vi "Create Sysdef Tree from DB Channel Clusters_BC.vi"(7 "Autocreate Rx timestamp chans?":bool, 8 "error in":errorcluster, 10 "BC":T1, 11 "Device Ptr":u64) -> (0 "error out":errorcluster, 3 "Device Ptr dup":u64)   [LabVIEW 2020, in "Ballard 1553 System Explorer.lvlib"]
uses:
  Ballard 1553 System Explorer.lvlib
  Parse XML Ballard/Ballard_BC.ctl
  Parse XML Ballard/Ballard_message.ctl
  Parse XML Ballard/Ballard_messageType.ctl
  Parse XML Ballard/Ballard_CWD1.ctl
  Parse XML Ballard/Ballard_CWD2.ctl
  Parse XML Ballard/Ballard_minorFrame.ctl
  Parse XML Ballard/Ballard_majorFrame.ctl
  Parse XML Ballard/Ballard_acyclicFrame.ctl
  <vilib>/NI VeriStand/Custom Device API/Custom Device Channel.ctl
  <vilib>/NI VeriStand/Custom Device API/Custom Device Channel Type.ctl
  Shared/Controls and Global/Global.vi
  <userlib>/_OpenG.lib/array/array.llb/Remove Duplicates from 1D Array (I32)__ogtk.vi
  <vilib>/NI VeriStand/Custom Device API/Set Item Property (String).vi
  <vilib>/NI VeriStand/Custom Device API/Set Item Property (U16).vi
  <vilib>/NI VeriStand/Custom Device API/Set Item Property (Variant).vi
  <vilib>/NI VeriStand/Custom Device API/Set Item Property (I32).vi
  <vilib>/NI VeriStand/Custom Device API/Custom Device API.lvlib
  Shared/Ballard 1553 Shared.lvlib
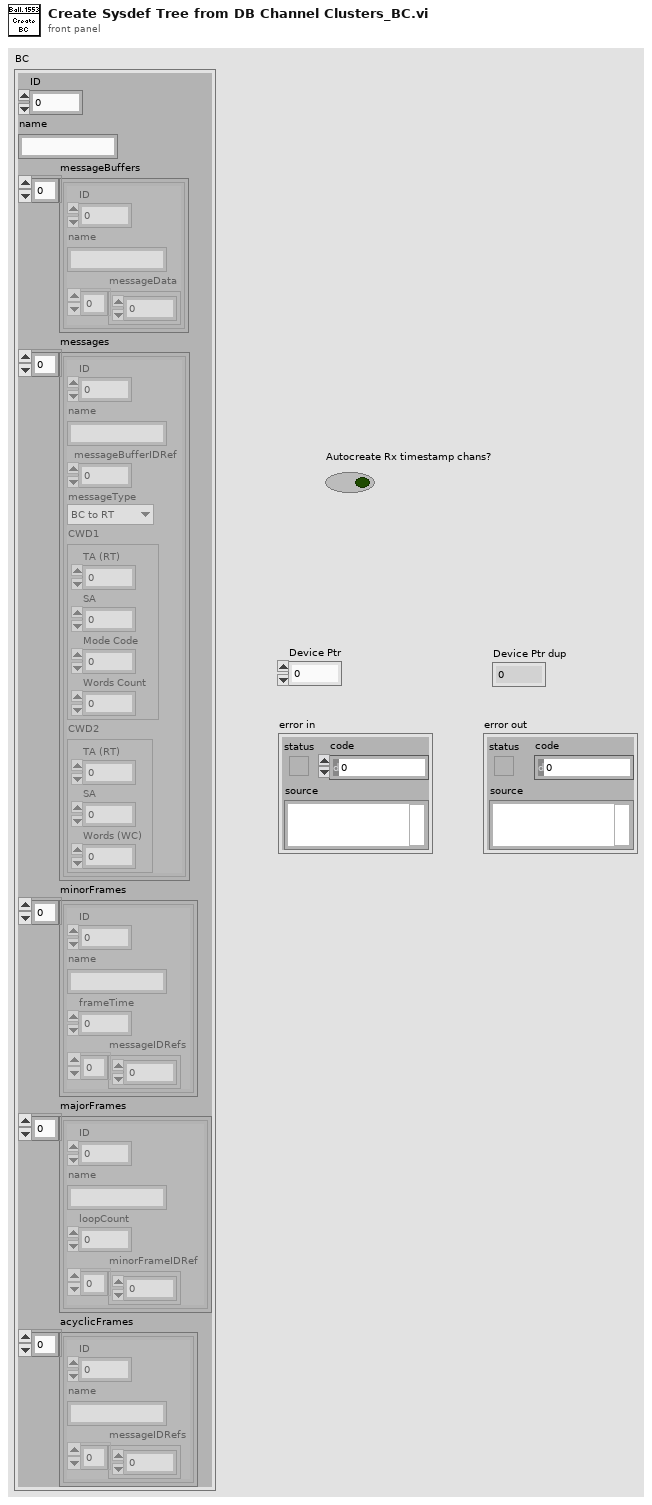
[diagram p1: front panel]
types:
  T1 = typedef "Ballard 1553 System Explorer.lvlib/Ballard_BC.ctl" = cluster{"ID":i32, "name":string, "messageBuffers":cluster{"ID":i32, "name":string, "messageData":u16[]}[], "messages":T2[], "minorFrames":T6[], "majorFrames":T7[], "acyclicFrames":T8[]}
  T2 = typedef "Ballard 1553 System Explorer.lvlib/Ballard_message.ctl" = cluster{"ID":i32, "name":string, "messageBufferIDRef":i32, "messageType":T3, "CWD1":T4, "CWD2":T5}
  T3 = typedef "Ballard 1553 System Explorer.lvlib/Ballard_messageType.ctl" = enum16{"BC to RT", "RT to BC", "RT to RT", "MC (Rx)", "MC (Tx)"}
  T4 = typedef "Ballard 1553 System Explorer.lvlib/Ballard_CWD1.ctl" = cluster{"TA (RT)":i8, "SA":i8, "Mode Code":i8, "Words Count":i8}
  T5 = typedef "Ballard 1553 System Explorer.lvlib/Ballard_CWD2.ctl" = cluster{"TA (RT)":i8, "SA":i8, "Words (WC)":i8}
  T6 = typedef "Ballard 1553 System Explorer.lvlib/Ballard_minorFrame.ctl" = cluster{"ID":i32, "name":string, "frameTime":i32, "messageIDRefs":i32[]}
  T7 = typedef "Ballard 1553 System Explorer.lvlib/Ballard_majorFrame.ctl" = cluster{"ID":i32, "name":string, "loopCount":i32, "minorFrameIDRef":i32[]}
  T8 = typedef "Ballard 1553 System Explorer.lvlib/Ballard_acyclicFrame.ctl" = cluster{"ID":i32, "name":string, "messageIDRefs":i32[]}
  T9 = typedef "Custom Device API.lvlib/Custom Device Channel.ctl" = cluster{"Type":T10, "Units":string, "Default Value":dbl, "Faultable":bool, "Scalable":bool}
  T10 = typedef "Custom Device API.lvlib/Custom Device Channel Type.ctl" = enum16{"Input", "Output"}
  T11 = cluster{"ID":i32, "name":string, "messageData":u16[]}[]
  T12 = typedef "Custom Device API.lvlib/Custom Device Item Ref.ctl" = u64
  T13 = cluster{"ID":i32, "name":string, "messageData":u16[]}
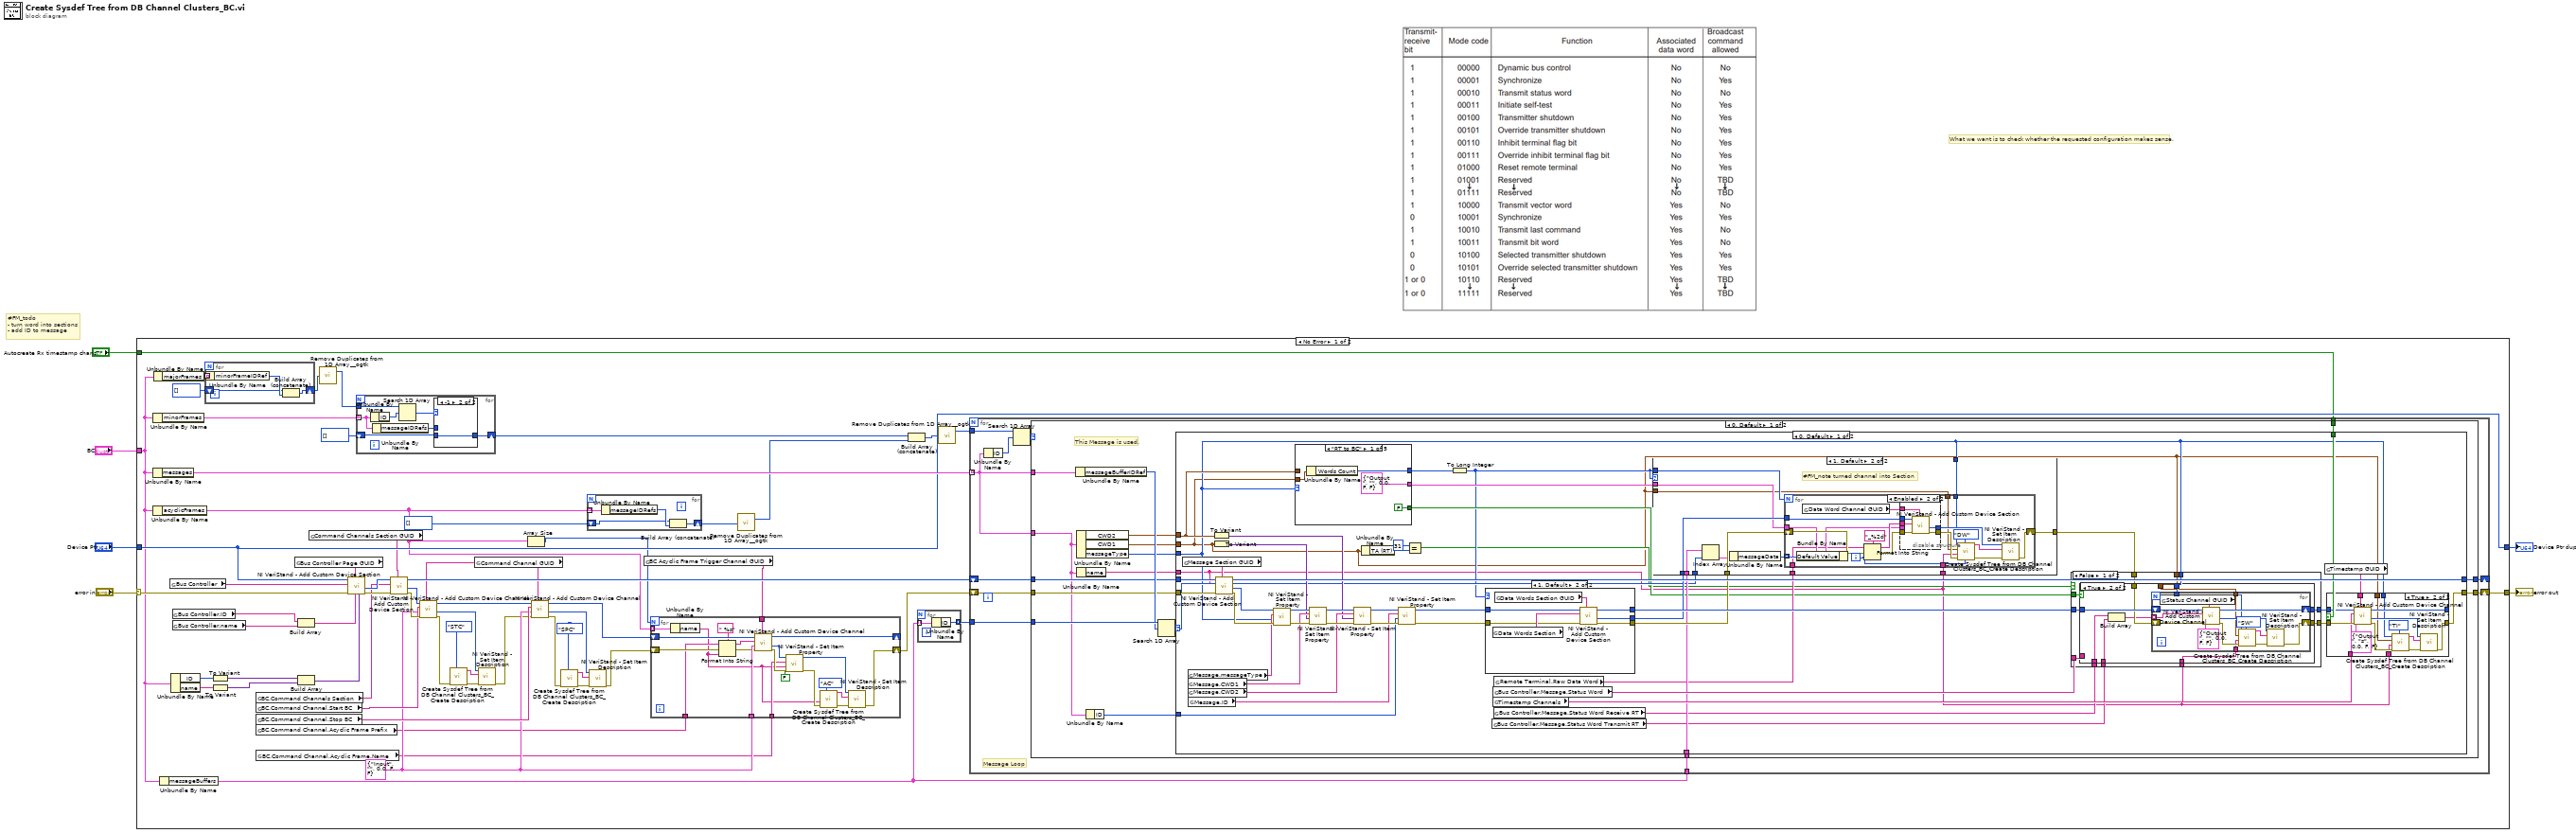
[diagram p0: block diagram]
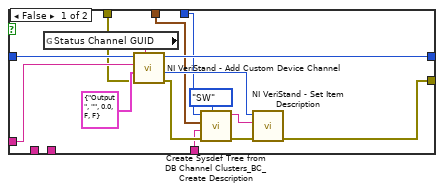
[diagram p2: hidden frame]
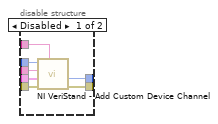
[diagram p6: hidden frame]
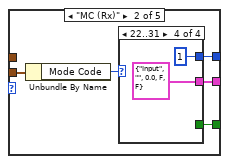
[diagram p7: hidden frame]
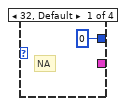
[diagram p8: hidden frame]
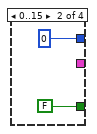
[diagram p9: hidden frame]
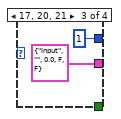
[diagram p10: hidden frame]
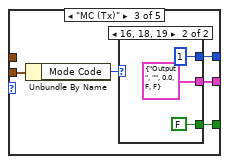
[diagram p11: hidden frame]
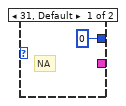
[diagram p12: hidden frame]
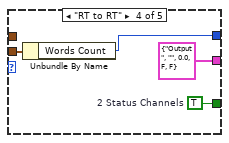
[diagram p13: hidden frame]
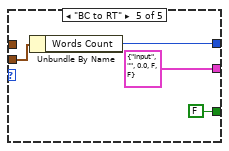
[diagram p14: hidden frame]
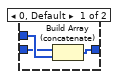
[diagram p18: hidden frame]
diagram:
  # "#FM_todo \n- turn word into sections\n- add ID to message"
  # "What we want is to check whether the requested configuration makes sense."
  n1 = case shown="No Error" "error in" {
    selector: "error in" -> [w67 w349]
    tunnel: [w49 w349] -> w5
    tunnel: "Device Ptr" -> [w50 w348]
    tunnel: [w50 w348] -> w3
    tunnel: "BC" -> [w34 _]
    tunnel: "Autocreate Rx timestamp chans?" -> [w46 _]
    frame No Error {
      w25 = T9 {"Type"=enum."Input", "Units"="", "Default Value"=0.0, "Faultable"=FALSE, "Scalable"=FALSE} ("Channel")
      n2 = Unbundle By Name(w34) -> ("minorFrames"=w57:T6[])
      n3 = Unbundle By Name(w34) -> ("messages"=w54:T2[])
      n4 = Unbundle By Name(w34) -> ("acyclicFrames"=w23:T8[])
      n5 = Unbundle By Name(w34) -> ("majorFrames"=w58:T7[])
      n6 = Unbundle By Name(w34) -> ("messageBuffers"=w52:T11)
      n7 = global read "Global.vi" "Bus Controller"() -> (w65:string)
      n8 = Unbundle By Name(w34) -> ("ID"=w64:i32, "name"=w63:string)
      n9 = global read "Global.vi" "Bus Controller.ID"() -> (w36:string)
      n10 = global read "Global.vi" "Bus Controller.name"() -> (w35:string)
      n11 = for {
        tunnel: w58 -> [w347] mode=indexing
        shift-right: [w346] -> w47
        shift-left: i32[] [] -> [w344]
        n12 = Unbundle By Name(w347) -> ("minorFrameIDRef"=w345:i32[])
        n13 = Build Array (concatenate)(w344, w345) -> (w346:i32[])
      }
      n14 = To Variant(anything=w64) -> (Variant=w62:variant)
      n15 = To Variant(anything=w63) -> (Variant=w61:variant)
      n16 = global read "Global.vi" "BC.Command Channels Section"() -> (w39:string)
      n17 = global read "Global.vi" "BC.Command Channel.Start BC"() -> (w38:string)
      n18 = global read "Global.vi" "BC.Command Channel.Stop BC"() -> (w37:string)
      n19 = global read "Global.vi" "BC.Command Channel.Acyclic Frame Prefix"() -> (w22:string)
      n20 = global read "Global.vi" "BC.Command Channel.Acyclic Frame.Name"() -> (w19:string)
      n21 = global read "Global.vi" "Bus Controller Page GUID"() -> (w66:string)
      n22 = Build Array(w36, w35) -> (w60:string[])
      n23 = Build Array(w62, w61) -> (w59:variant[])
      n24 = global read "Global.vi" "Command Channels Section GUID"() -> (w20:string)
      n25 = call-poly <userlib>:"Remove Duplicates from 1D Array__ogtk.vi"("Input Array"=w47) -> ("Output Array"=w56:i32[])  [unwired: 1 out]
      n26 = call <vilib>:"NI VeriStand - Add Custom Device Section.vi"("Property Values"=w59, "Property names"=w60, "GUID (Default Section)"=w66, "error in (no error)"=w67, "Section Name"=w65, "Parent Ref in"=w50) -> ("error out"=w40:errorcluster, "Section Ptr"=w42:T12)  [unwired: 2 in, 2 out]
      n27 = for {
        tunnel: w57 -> [w336] mode=indexing
        tunnel: w56 -> [w339]
        shift-right: [w334] -> w31
        shift-left: i32[] [] -> [w333]
        n28 = Unbundle By Name(w336) -> ("ID"=w338:i32)
        n29 = Unbundle By Name(w336) -> ("messageIDRefs"=w335:i32[])
        n30 = Search 1D Array(1D array=w339, element=w338) -> (index of element=w337:i32)  [unwired: 1 in]
        n31 = case shown="-1" w337 {
          tunnel: w335 -> [w342 _]
          tunnel: [w341 w343] -> w334
          tunnel: w333 -> [w340 w343]
          frame 0, Default {
            n32 = Build Array (concatenate)(w340, w342) -> (w341:i32[])
          }
          frame -1 {
          }
        }
      }
      n33 = call <vilib>:"NI VeriStand - Add Custom Device Section.vi"("GUID (Default Section)"=w20, "error in (no error)"=w40, "Section Name"=w39, "Parent Ref in"=w42) -> ("error out"=w44:errorcluster, "Section Ptr"=w43:T12, "Parent Ref out"=w41:T12)  [unwired: 4 in, 1 out]
      n34 = global read "Global.vi" "Command Channel GUID"() -> (w27:string)
      n35 = call <vilib>:"NI VeriStand - Add Custom Device Channel.vi"("GUID (Default Channel)"=w27, "error in (no error)"=w44, "Channel"=w25, "Channel Name"=w38, "Parent Ref in"=w43) -> ("error out"=w17:errorcluster, "Channel Ref"=w16:T12, "Parent Ref out"=w45:T12)  [unwired: 3 in, 1 out]
      n36 = call "Create Sysdef Tree from DB Channel Clusters_BC_Create Description.vi"("Type"=enum16{"DW", "STC", "SPC", "SW", "TI", "AC"}."STC", "error in (no error)"=w17) -> ("error out"=w14:errorcluster, "Description (Out)"=w18:string)  [unwired: 8 in]
      n37 = call <vilib>:"NI VeriStand - Set Item Description.vi"("error in (no error)"=w14, "Description"=w18, "Item Ref in"=w16) -> ("error out"=w15:errorcluster)  [unwired: 6 in, 2 out]
      n38 = Array Size(array=w23) -> (size(s)=w26:i32)
      n39 = call <vilib>:"NI VeriStand - Add Custom Device Channel.vi"("GUID (Default Channel)"=w27, "error in (no error)"=w15, "Channel"=w25, "Channel Name"=w37, "Parent Ref in"=w45) -> ("error out"=w10:errorcluster, "Channel Ref"=w8:T12, "Parent Ref out"=w24:T12)  [unwired: 3 in, 1 out]
      n40 = call "Create Sysdef Tree from DB Channel Clusters_BC_Create Description.vi"("Type"=enum16{"DW", "STC", "SPC", "SW", "TI", "AC"}."SPC", "error in (no error)"=w10) -> ("error out"=w12:errorcluster, "Description (Out)"=w11:string)  [unwired: 8 in]
      n41 = for {
        tunnel: w23 -> [w92] mode=indexing
        shift-right: [w90] -> w32
        shift-left: i32[] [] -> [w89]
        n42 = Unbundle By Name(w92) -> ("messageIDRefs"=w91:i32[])
        n43 = Build Array (concatenate)(w89, w91) -> (w90:i32[])
      }
      n44 = call <vilib>:"NI VeriStand - Set Item Description.vi"("error in (no error)"=w12, "Description"=w11, "Item Ref in"=w8) -> ("error out"=w9:errorcluster)  [unwired: 6 in, 2 out]
      n45 = global read "Global.vi" "BC Acyclic Frame Trigger Channel GUID"() -> (w21:string)
      n46 = for {
        N: w26 -> [_]
        shift-right: [w71] -> w28
        shift-left: w9 -> [w84]
        tunnel: w21 -> [w88]
        tunnel: w25 -> [w87]
        shift-right: [w85] -> _
        shift-left: w24 -> [w86]
        tunnel: w23 -> [w82] mode=indexing
        tunnel: w22 -> [w81]
        tunnel: w19 -> [w75]
        n47 = Unbundle By Name(w82) -> ("name"=w68:string)
        n48 = Format Into String(format string=" %s", initial string=w81, error in=w84, w68) -> (resulting string=w79:string, error out=w83:errorcluster)
        n49 = call <vilib>:"NI VeriStand - Add Custom Device Channel.vi"("GUID (Default Channel)"=w88, "error in (no error)"=w83, "Channel"=w87, "Channel Name"=w79, "Parent Ref in"=w86) -> ("error out"=w76:errorcluster, "Channel Ref"=w78:T12, "Parent Ref out"=w85:T12)  [unwired: 3 in, 1 out]
        n50 = call-poly <vilib>:"NI VeriStand - Set Item Property.vi"("Binary String (T)"=FALSE, "error in (no error)"=w76, "Value"=w68, "Property Name"=w75, "Item Ref in"=w78) -> ("error out"=w69:errorcluster, "Item Ref out"=w70:T12)  [unwired: 4 in, 1 out]
        n51 = call "Create Sysdef Tree from DB Channel Clusters_BC_Create Description.vi"("Type"=enum16{"DW", "STC", "SPC", "SW", "TI", "AC"}."AC", "error in (no error)"=w69, "Message Name"=w68) -> ("error out"=w73:errorcluster, "Description (Out)"=w72:string)  [unwired: 7 in]
        n52 = call <vilib>:"NI VeriStand - Set Item Description.vi"("error in (no error)"=w73, "Description"=w72, "Item Ref in"=w70) -> ("error out"=w71:errorcluster)  [unwired: 6 in, 2 out]
      }
      n53 = call-poly <userlib>:"Remove Duplicates from 1D Array__ogtk.vi"("Input Array"=w32) -> ("Output Array"=w30:i32[])  [unwired: 1 out]
      n54 = Build Array (concatenate)(w31, w30) -> (w29:i32[])
      n55 = for {
        tunnel: w52 -> [w94] mode=indexing
        tunnel: [w93] -> w51 mode=indexing
        n56 = Unbundle By Name(w94) -> ("ID"=w93:i32)
      }
      n57 = call-poly <userlib>:"Remove Duplicates from 1D Array__ogtk.vi"("Input Array"=w29) -> ("Output Array"=w53:i32[])  [unwired: 1 out]
      n58 = for {
        tunnel: w54 -> [w97] mode=indexing
        tunnel: w53 -> [w105]
        tunnel: w52 -> [w100]
        tunnel: w51 -> [w99]
        shift-right: [w96] -> _
        shift-left: w41 -> [w102]
        shift-right: [w98] -> w49
        shift-left: w28 -> [w101]
        tunnel: w46 -> [w95]
        # "Message Loop"
        n59 = Unbundle By Name(w97) -> ("ID"=w104:i32)
        n60 = Search 1D Array(1D array=w105, element=w104) -> (index of element=w103:i32)  [unwired: 1 in]
        n61 = case shown="0, Default" w103 {
          tunnel: w97 -> [w121 _]
          tunnel: w102 -> [w115 w331]
          tunnel: w101 -> [w116 w332]
          tunnel: w100 -> [w117 _]
          tunnel: w99 -> [w120 _]
          tunnel: [w114 w332] -> w98
          tunnel: w97 -> [w107 _]
          tunnel: [w112 w331] -> w96
          tunnel: w95 -> [w111 _]
          frame 0, Default {
            # "This Message is used."
            n62 = Unbundle By Name(w121) -> ("messageBufferIDRef"=w119:i32)
            n63 = Unbundle By Name(w107) -> ("CWD2"=w109:T5, "CWD1"=w110:T4, "messageType"=w108:T3)
            n64 = Unbundle By Name(w107) -> ("name"=w113:string)
            n65 = Unbundle By Name(w107) -> ("ID"=w106:i32)
            n66 = Search 1D Array(1D array=w120, element=w119) -> (index of element=w118:i32)  [unwired: 1 in]
            n67 = case shown="0, Default" w118 {
              selector: w118 -> [w140 _]
              tunnel: w117 -> [w141 _]
              tunnel: w116 -> [w169 w330]
              tunnel: w115 -> [w168 w329]
              tunnel: [w139 w330] -> w114
              tunnel: w113 -> [w125 _]
              tunnel: [w167 w329] -> w112
              tunnel: w111 -> [w162 _]
              tunnel: w110 -> [w126 _]
              tunnel: w109 -> [w147 _]
              tunnel: w108 -> [w127 _]
              tunnel: w106 -> [w122 _]
              frame 0, Default {
                n68 = global read "Global.vi" "Message Section GUID"() -> (w159:string)
                n69 = global read "Global.vi" "Message.messageType"() -> (w156:string)
                n70 = global read "Global.vi" "Message.CWD1"() -> (w151:string)
                n71 = global read "Global.vi" "Message.CWD2"() -> (w149:string)
                n72 = global read "Global.vi" "Message.ID"() -> (w131:string)
                n73 = To Variant(anything=w147) -> (Variant=w148:variant)
                n74 = To Variant(anything=w126) -> (Variant=w150:variant)
                n75 = call <vilib>:"NI VeriStand - Add Custom Device Section.vi"("GUID (Default Section)"=w159, "error in (no error)"=w169, "Section Name"=w125, "Parent Ref in"=w168) -> ("error out"=w157:errorcluster, "Section Ptr"=w158:T12, "Parent Ref out"=w167:T12)  [unwired: 4 in, 1 out]
                n76 = call-poly <vilib>:"NI VeriStand - Set Item Property.vi"("error in (no error)"=w157, "Value"=w127, "Property Name"=w156, "Item Ref in"=w158) -> ("error out"=w155:errorcluster, "Item Ref out"=w152:T12)  [unwired: 5 in, 1 out]
                n77 = case shown="\"RT to BC\"" w127 {
                  tunnel: w147 -> [_ _ _ _ _]
                  tunnel: w126 -> [w280 w285 w297 w306 w309]
                  tunnel: [w282 w287 w299 w305 w311] -> w146
                  tunnel: [T9 {"Type"=enum."Output", "Units"="", "Default Value"=0.0, "Faultable"=FALSE, "Scalable"=FALSE} ("Channel") w283 w295 T9 {"Type"=enum."Output", "Units"="", "Default Value"=0.0, "Faultable"=FALSE, "Scalable"=FALSE} ("Channel") T9 {"Type"=enum."Input", "Units"="", "Default Value"=0.0, "Faultable"=FALSE, "Scalable"=FALSE} ("Channel")] -> w144
                  tunnel: [FALSE ("2 Status Channels") w286 w298 w307 FALSE ("2 Status Channels")] -> w137
                  frame "RT to BC" {
                    n78 = Unbundle By Name(w280) -> ("Words Count"=w282:i8)
                  }
                  frame "MC (Rx)" {
                    n79 = Unbundle By Name(w285) -> ("Mode Code"=w284:i8)
                    n80 = case shown="22..31" w284 {
                      tunnel: [i8 0 ("Words (WC)") i8 0 ("Words (WC)") i8 1 ("Words (WC)") i8 1 ("Words (WC)")] -> w287
                      tunnel: [_ FALSE ("2 Status Channels") _ _] -> w286
                      tunnel: [_ _ T9 {"Type"=enum."Input", "Units"="", "Default Value"=0.0, "Faultable"=FALSE, "Scalable"=FALSE} ("Channel") T9 {"Type"=enum."Input", "Units"="", "Default Value"=0.0, "Faultable"=FALSE, "Scalable"=FALSE} ("Channel")] -> w283
                      frame 32, Default {
                        # "NA"
                      }
                      frame 0..15 {
                      }
                      frame 17, 20, 21 {
                      }
                      frame 22..31 {
                      }
                    }
                  }
                  frame "MC (Tx)" {
                    n81 = Unbundle By Name(w297) -> ("Mode Code"=w296:i8)
                    n82 = case shown="16, 18, 19" w296 {
                      tunnel: [i8 0 ("Words (WC)") i8 1 ("Words (WC)")] -> w299
                      tunnel: [_ FALSE ("2 Status Channels")] -> w298
                      tunnel: [_ T9 {"Type"=enum."Output", "Units"="", "Default Value"=0.0, "Faultable"=FALSE, "Scalable"=FALSE} ("Channel")] -> w295
                      frame 31, Default {
                        # "NA"
                      }
                      frame 16, 18, 19 {
                      }
                    }
                  }
                  frame "RT to RT" {
                    w307 = TRUE  # 2 Status Channels
                    n83 = Unbundle By Name(w306) -> ("Words Count"=w305:i8)
                  }
                  frame "BC to RT" {
                    n84 = Unbundle By Name(w309) -> ("Words Count"=w311:i8)
                  }
                }
                n85 = call-poly <vilib>:"NI VeriStand - Set Item Property.vi"("error in (no error)"=w155, "Value"=w150, "Property Name"=w151, "Item Ref in"=w152) -> ("error out"=w154:errorcluster, "Item Ref out"=w153:T12)  [unwired: 5 in, 1 out]
                n86 = call-poly <vilib>:"NI VeriStand - Set Item Property.vi"("error in (no error)"=w154, "Value"=w148, "Property Name"=w149, "Item Ref in"=w153) -> ("error out"=w132:errorcluster, "Item Ref out"=w133:T12)  [unwired: 5 in, 1 out]
                n87 = Unbundle By Name(w126) -> ("TA (RT)"=w130:i8)
                n88 = call-poly <vilib>:"NI VeriStand - Set Item Property.vi"("error in (no error)"=w132, "Value"=w122, "Property Name"=w131, "Item Ref in"=w133) -> ("error out"=w123:errorcluster, "Item Ref out"=w124:T12)  [unwired: 5 in, 1 out]
                n89 = Equal?(x=i8 31, y=w130) -> (x = y?=w128:bool)
                n90 = To Long Integer(number=w146) -> (32bit integer=w134:i32)
                n91 = case shown="1, Default" w134 {
                  tunnel: [w224 w230] -> w166
                  tunnel: w123 -> [w223 w229]
                  tunnel: w124 -> [w224 w228]
                  tunnel: [_ w227] -> w145
                  tunnel: [w223 w226] -> w143
                  frame 0 {
                    # "No Data Words to be created\nWe don't create the Section"
                  }
                  frame 1, Default {
                    n92 = global read "Global.vi" "Data Words Section"() -> (w231:string)
                    n93 = global read "Global.vi" "Data Words Section GUID"() -> (w225:string)
                    n94 = call <vilib>:"NI VeriStand - Add Custom Device Section.vi"("GUID (Default Section)"=w225, "error in (no error)"=w229, "Section Name"=w231, "Parent Ref in"=w228) -> ("error out"=w226:errorcluster, "Section Ptr"=w227:T12, "Parent Ref out"=w230:T12)  [unwired: 4 in, 1 out]
                  }
                }
                n95 = global read "Global.vi" "Bus Controller.Message.Status Word Transmit RT"() -> (w135:string)
                n96 = global read "Global.vi" "Bus Controller.Message.Status Word"() -> (w165:string)
                n97 = global read "Global.vi" "Timestamp Channels"() -> (w160:string)
                n98 = global read "Global.vi" "Bus Controller.Message.Status Word Receive RT"() -> (w136:string)
                n99 = global read "Global.vi" "Remote Terminal.Raw Data Word"() -> (w138:string)
                n100 = case shown="1, Default" w134 {
                  tunnel: w134 -> [_ w245]
                  tunnel: w145 -> [_ w244]
                  tunnel: w144 -> [_ w243]
                  tunnel: w143 -> [w232 w242]
                  tunnel: [w232 w241] -> w142
                  tunnel: w141 -> [_ w240]
                  tunnel: w140 -> [_ w239]
                  tunnel: w138 -> [_ w236]
                  tunnel: w125 -> [_ w235]
                  tunnel: w126 -> [_ w234]
                  tunnel: w127 -> [_ w233]
                  frame 0 {
                    # "No Data Words to be created"
                  }
                  frame 1, Default {
                    # "#FM_note turned channel into Section"
                    n101 = Index Array(array=w240, index=w239) -> (element=w238:T13)
                    n102 = Unbundle By Name(w238) -> ("messageData"=w237:u16[])
                    n103 = for {
                      N: w245 -> [_]
                      tunnel: w244 -> [w265]
                      tunnel: w243 -> [w260]
                      shift-right: [w254] -> w241
                      shift-left: w242 -> [w263]
                      tunnel: w237 -> [w258] mode=indexing
                      tunnel: w236 -> [w256]
                      tunnel: w235 -> [w249]
                      tunnel: w234 -> [w248]
                      tunnel: w233 -> [w247]
                      i -> [w250]
                      n104 = Bundle By Name(cluster=w260, "Default Value"=w258) -> (w259:T9)
                      n105 = global read "Global.vi" "Data Word Channel GUID"() -> (w257:string)
                      n106 = Format Into String(format string="_%2d", initial string=w256, error in=w263, w250) -> (resulting string=w261:string, error out=w262:errorcluster)
                      n107 = disable-structure shown="Enabled" {
                        disable-tunnel: w265 -> [w272 w275]
                        disable-tunnel: w262 -> [w271 w277]
                        disable-tunnel: w261 -> [w270 w273]
                        disable-tunnel: w259 -> [w269 _]
                        disable-tunnel: w257 -> [w268 w274]
                        disable-tunnel: [w267 w276] -> w255
                        disable-tunnel: [w266 w278] -> w253
                        frame Disabled {
                          n108 = call <vilib>:"NI VeriStand - Add Custom Device Channel.vi"("GUID (Default Channel)"=w268, "error in (no error)"=w271, "Channel"=w269, "Channel Name"=w270, "Parent Ref in"=w272) -> ("error out"=w266:errorcluster, "Channel Ref"=w267:T12)  [unwired: 3 in, 2 out]
                        }
                        frame Enabled {
                          n109 = call <vilib>:"NI VeriStand - Add Custom Device Section.vi"("GUID (Default Section)"=w274, "error in (no error)"=w277, "Section Name"=w273, "Parent Ref in"=w275) -> ("error out"=w278:errorcluster, "Section Ptr"=w276:T12)  [unwired: 4 in, 2 out]
                        }
                      }
                      n110 = call "Create Sysdef Tree from DB Channel Clusters_BC_Create Description.vi"("Word Index"=w250, "Type"=enum16{"DW", "STC", "SPC", "SW", "TI", "AC"}."DW", "error in (no error)"=w253, "Message Name"=w249, "CWD1"=w248, "messageType"=w247) -> ("error out"=w252:errorcluster, "Description (Out)"=w251:string)  [unwired: 4 in]
                      n111 = call <vilib>:"NI VeriStand - Set Item Description.vi"("error in (no error)"=w252, "Description"=w251, "Item Ref in"=w255) -> ("error out"=w254:errorcluster)  [unwired: 6 in, 2 out]
                    }
                  }
                }
                n112 = case shown="False" w128 {
                  tunnel: w166 -> [w180 w222]
                  tunnel: w165 -> [w179 _]
                  tunnel: [w178 w222] -> w164
                  tunnel: [w177 w221] -> w163
                  tunnel: w142 -> [w176 w221]
                  tunnel: w137 -> [w175 _]
                  tunnel: w136 -> [w174 _]
                  tunnel: w135 -> [w173 _]
                  tunnel: w127 -> [w172 _]
                  tunnel: w126 -> [w171 _]
                  tunnel: w125 -> [w170 _]
                  frame False {
                    n113 = case shown="True" w175 {
                      tunnel: w180 -> [w195 w205]
                      tunnel: w179 -> [w194 _]
                      tunnel: [w193 w204] -> w178
                      tunnel: [w184 w203] -> w177
                      tunnel: w176 -> [w191 w202]
                      tunnel: w174 -> [_ w201]
                      tunnel: w173 -> [_ w200]
                      tunnel: w172 -> [w183 w198]
                      tunnel: w171 -> [w182 w197]
                      tunnel: w170 -> [w181 w196]
                      frame False {
                        n114 = global read "Global.vi" "Status Channel GUID"() -> (w190:string)
                        n115 = call <vilib>:"NI VeriStand - Add Custom Device Channel.vi"("GUID (Default Channel)"=w190, "error in (no error)"=w191, "Channel"=T9 {"Type"=enum."Output", "Units"="", "Default Value"=0.0, "Faultable"=FALSE, "Scalable"=FALSE}, "Channel Name"=w194, "Parent Ref in"=w195) -> ("error out"=w187:errorcluster, "Channel Ref"=w185:T12, "Parent Ref out"=w193:T12)  [unwired: 3 in, 1 out]
                        n116 = call "Create Sysdef Tree from DB Channel Clusters_BC_Create Description.vi"("Type"=enum16{"DW", "STC", "SPC", "SW", "TI"}."SW", "error in (no error)"=w187, "Message Name"=w181, "CWD1"=w182, "messageType"=w183) -> ("error out"=w186:errorcluster, "Description (Out)"=w188:string)  [unwired: 5 in]
                        n117 = call <vilib>:"NI VeriStand - Set Item Description.vi"("error in (no error)"=w186, "Description"=w188, "Item Ref in"=w185) -> ("error out"=w184:errorcluster)  [unwired: 6 in, 2 out]
                      }
                      frame True {
                        n118 = Build Array(w201, w200) -> (w199:string[])
                        n119 = for {
                          shift-right: [w219] -> w204
                          shift-left: w205 -> [w220]
                          shift-right: [w211] -> w203
                          shift-left: w202 -> [w217]
                          tunnel: w199 -> [w215] mode=indexing
                          tunnel: w198 -> [w209]
                          tunnel: w197 -> [w208]
                          tunnel: w196 -> [w207]
                          n120 = global read "Global.vi" "Status Channel GUID"() -> (w216:string)
                          n121 = call <vilib>:"NI VeriStand - Add Custom Device Channel.vi"("GUID (Default Channel)"=w216, "error in (no error)"=w217, "Channel"=T9 {"Type"=enum."Output", "Units"="", "Default Value"=0.0, "Faultable"=FALSE, "Scalable"=FALSE}, "Channel Name"=w215, "Parent Ref in"=w220) -> ("error out"=w212:errorcluster, "Channel Ref"=w210:T12, "Parent Ref out"=w219:T12)  [unwired: 3 in, 1 out]
                          n122 = call "Create Sysdef Tree from DB Channel Clusters_BC_Create Description.vi"("Type"=enum16{"DW", "STC", "SPC", "SW", "TI", "AC"}."SW", "error in (no error)"=w212, "Message Name"=w207, "CWD1"=w208, "messageType"=w209) -> ("error out"=w214:errorcluster, "Description (Out)"=w213:string)  [unwired: 5 in]
                          n123 = call <vilib>:"NI VeriStand - Set Item Description.vi"("error in (no error)"=w214, "Description"=w213, "Item Ref in"=w210) -> ("error out"=w211:errorcluster)  [unwired: 6 in, 2 out]
                        }
                      }
                    }
                  }
                  frame True {
                  }
                }
                n124 = global read "Global.vi" "Timestamp GUID"() -> (w161:string)
                n125 = case shown="True" w162 {
                  tunnel: w164 -> [w312 w328]
                  tunnel: w163 -> [w313 w327]
                  tunnel: [w313 w318] -> w139
                  tunnel: [w312 w325] -> _
                  tunnel: w161 -> [_ w326]
                  tunnel: w160 -> [_ w324]
                  tunnel: w127 -> [_ w317]
                  tunnel: w126 -> [_ w316]
                  tunnel: w125 -> [_ w315]
                  frame False {
                  }
                  frame True {
                    n126 = call <vilib>:"NI VeriStand - Add Custom Device Channel.vi"("GUID (Default Channel)"=w326, "error in (no error)"=w327, "Channel"=T9 {"Type"=enum."Output", "Units"="s", "Default Value"=0.0, "Faultable"=FALSE, "Scalable"=FALSE}, "Channel Name"=w324, "Parent Ref in"=w328) -> ("error out"=w320:errorcluster, "Channel Ref"=w319:T12, "Parent Ref out"=w325:T12)  [unwired: 3 in, 1 out]
                    n127 = call "Create Sysdef Tree from DB Channel Clusters_BC_Create Description.vi"("Type"=enum16{"DW", "STC", "SPC", "SW", "TI", "AC"}."TI", "error in (no error)"=w320, "Message Name"=w315, "CWD1"=w316, "messageType"=w317) -> ("error out"=w321:errorcluster, "Description (Out)"=w322:string)  [unwired: 5 in]
                    n128 = call <vilib>:"NI VeriStand - Set Item Description.vi"("error in (no error)"=w321, "Description"=w322, "Item Ref in"=w319) -> ("error out"=w318:errorcluster)  [unwired: 6 in, 2 out]
                  }
                }
              }
              frame -1 {
              }
            }
          }
          frame -1 {
          }
        }
      }
    }
    frame Error {
    }
  }
  "error out" <- w5
  "Device Ptr dup" <- w3
